vi "ZK_TriggerMouse.vi"(8 "Cluster 3":cluster{"X1":i32, "Y1":i32, "X2":i32, "Y2":i32}={"X1"=1479, "Y1"=207, "X2"=1532, "Y2"=259}, 10 "Result":T1={"A_Row"=2, "A_Col"=0, "B_Row"=1, "B_Col"=0}) -> ()   [LabVIEW 2018]
uses:
  <vilib>/Utility/error.llb/DialogType.ctl
  C:/Users/rshang/Desktop/LabVIEWZOOKEPPER_V2/ClassLibrary_ZK.dll
  ClassLibrary_ZK.dll
panel:
  out "String 2":string
  out "String":string
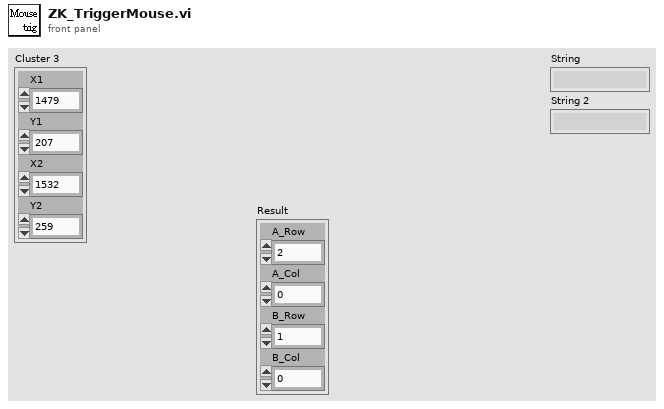
[diagram p1: front panel]
types:
  T1 = cluster{"A_Row":i32, "A_Col":i32, "B_Row":i32, "B_Col":i32}
  T2 = typedef "DialogType.ctl" = u16
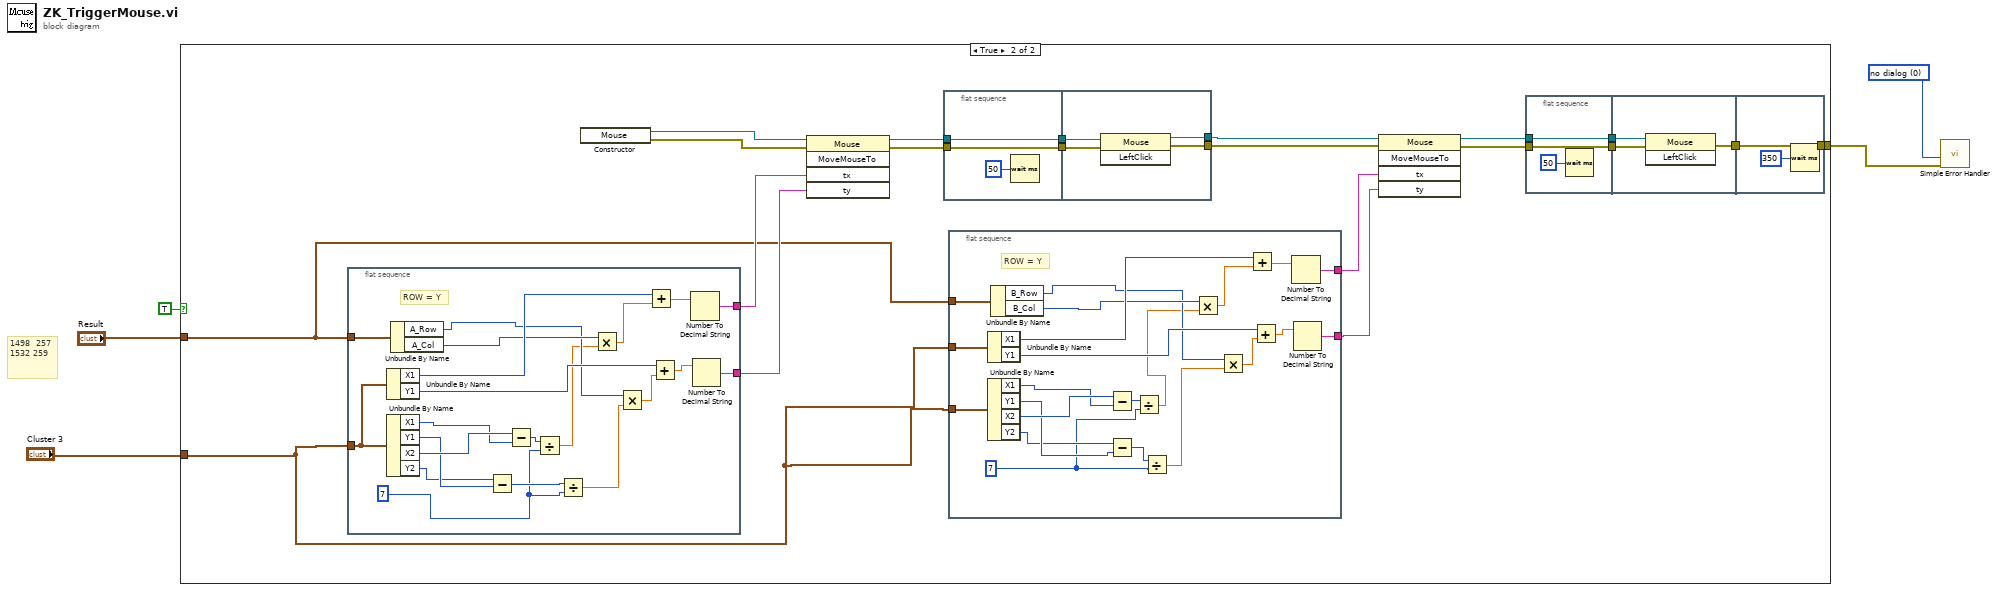
[diagram p0: block diagram]
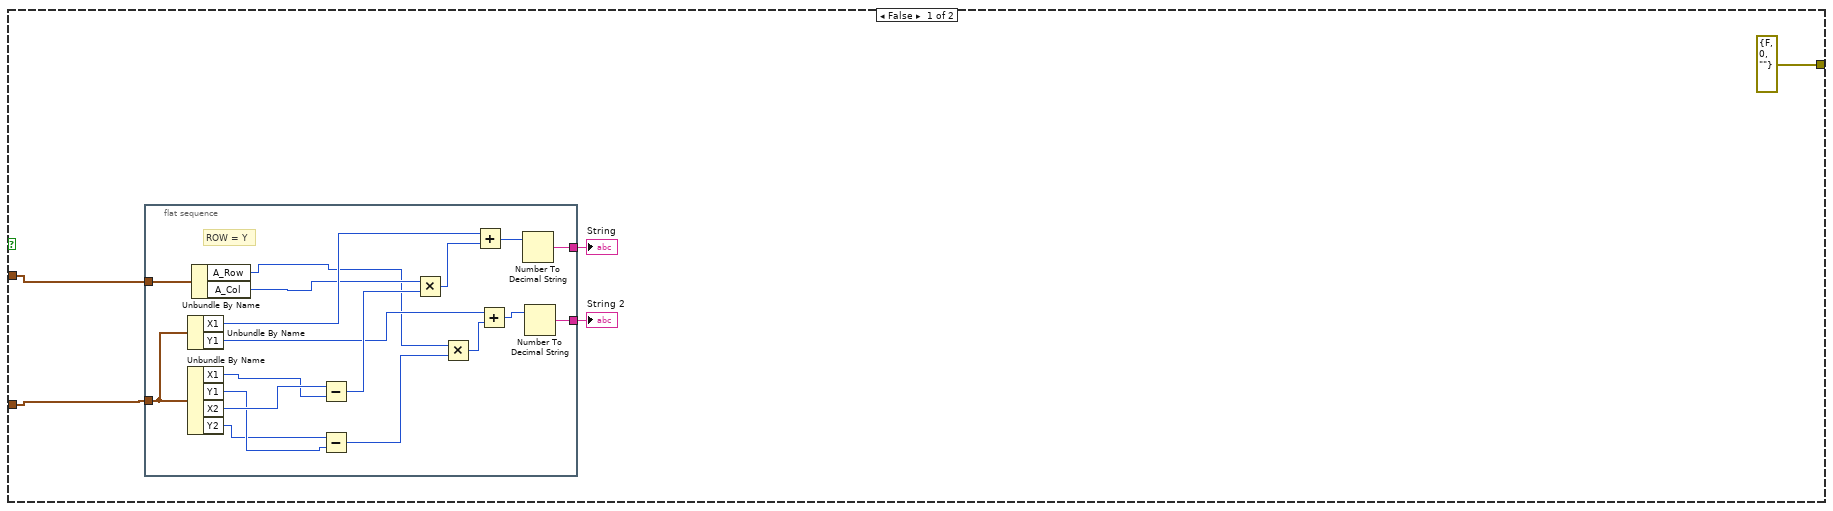
[diagram p2: hidden frame]
diagram:
  w1 = T2 0 items=["no dialog", "OK message", "continue or stop message", "OK message + warnings", "continue/stop + warnings"] ("type of dialog (OK msg:1)")
  # "1498  257 \n1532 259"
  n1 = case shown="True" TRUE {
    tunnel: "Result" -> [w10 w38]
    tunnel: "Cluster 3" -> [w9 w35]
    tunnel: [errorcluster {"status"=FALSE, "code"=0, "source"=""} ("error out") w30] -> w2
    frame False {
      n2 = flat-sequence {
        tunnel: [w16] -> w7
        tunnel: [w15] -> w8
        tunnel: w10 -> [w12]
        tunnel: w9 -> [w11]
        frame #0 {
          # "ROW = Y"
          n3 = Unbundle By Name(w11) -> ("X1"=w24:i32, "Y1"=w21:i32)
          n4 = Unbundle By Name(w11) -> ("X1"=w27:i32, "Y1"=w26:i32, "X2"=w28:i32, "Y2"=w25:i32)
          n5 = Unbundle By Name(w12) -> ("A_Row"=w13:i32, "A_Col"=w14:i32)
          n6 = Subtract(x=w28, y=w27) -> (x-y=w23:i32)
          n7 = Subtract(x=w25, y=w26) -> (x-y=w20:i32)
          n8 = Multiply(x=w14, y=w23) -> (x*y=w22:i32)
          n9 = Multiply(x=w13, y=w20) -> (x*y=w19:i32)
          n10 = Add(x=w24, y=w22) -> (x+y=w18:i32)
          n11 = Add(x=w21, y=w19) -> (x+y=w17:i32)
          n12 = Number To Decimal String(number=w18) -> (decimal integer string=w15:string)  [unwired: 1 in]
          n13 = Number To Decimal String(number=w17) -> (decimal integer string=w16:string)  [unwired: 1 in]
        }
      }
      "String" <- w8
      "String 2" <- w7
    }
    frame True {
      n14 = flat-sequence {
        tunnel: [w95] -> w46
        tunnel: [w94] -> w45
        tunnel: w38 -> [w91]
        tunnel: w35 -> [w90]
        frame #0 {
          w86 = 7 ("y")
          # "ROW = Y"
          n15 = Unbundle By Name(w90) -> ("X1"=w101:i32, "Y1"=w99:i32)
          n16 = Unbundle By Name(w90) -> ("X1"=w104:i32, "Y1"=w103:i32, "X2"=w105:i32, "Y2"=w102:i32)
          n17 = Unbundle By Name(w91) -> ("A_Row"=w92:i32, "A_Col"=w93:i32)
          n18 = Subtract(x=w102, y=w103) -> (x-y=w87:i32)
          n19 = Subtract(x=w105, y=w104) -> (x-y=w89:i32)
          n20 = Divide(x=w89, y=w86) -> (x/y=w88:dbl)
          n21 = Divide(x=w87, y=w86) -> (x/y=w85:dbl)
          n22 = Multiply(x=w93, y=w88) -> (x*y=w100:dbl)
          n23 = Multiply(x=w92, y=w85) -> (x*y=w98:dbl)
          n24 = Add(x=w101, y=w100) -> (x+y=w97:dbl)
          n25 = Add(x=w99, y=w98) -> (x+y=w96:dbl)
          n26 = Number To Decimal String(number=w97) -> (decimal integer string=w94:string)  [unwired: 1 in]
          n27 = Number To Decimal String(number=w96) -> (decimal integer string=w95:string)  [unwired: 1 in]
        }
      }
      n28 = constructor class="Mouse"() -> (reference out=w48:refnum<k24>, error out=w47:errorcluster)  [unwired: 3 in, 1 out]
      n29 = invoke class="Mouse" method="MoveMouseTo"(reference=w48, error in=w47, "tx"=w45, "ty"=w46) -> (reference out=w44:refnum<k24>, error out=w43:errorcluster)  [unwired: 1 in, 3 out]
      n30 = flat-sequence {
        tunnel: w43 -> [w58]
        tunnel: w44 -> [w59]
        tunnel: [w59] -> w34
        tunnel: [w58] -> w33
        tunnel: [w61] -> w42
        tunnel: [w60] -> w40
        tunnel: w34 -> [w63]
        tunnel: w33 -> [w62]
        frame #0 {
          n31 = Wait (ms)(milliseconds to wait=u32 50) -> ()  [unwired: 1 out]
        }
        frame #1 {
          n32 = invoke class="Mouse" method="LeftClick"(reference=w63, error in=w62) -> (reference out=w61:refnum<k24>, error out=w60:errorcluster)  [unwired: 1 in, 1 out]
        }
      }
      n33 = flat-sequence {
        tunnel: [w74] -> w36
        tunnel: [w73] -> w37
        tunnel: w38 -> [w70]
        tunnel: [w69] -> _
        tunnel: w35 -> [w69]
        tunnel: w35 -> [_]
        frame #0 {
          w65 = 7 ("y")
          # "ROW = Y"
          n34 = Unbundle By Name(w69) -> ("X1"=w80:i32, "Y1"=w78:i32)
          n35 = Unbundle By Name(w69) -> ("X1"=w83:i32, "Y1"=w82:i32, "X2"=w84:i32, "Y2"=w81:i32)
          n36 = Unbundle By Name(w70) -> ("B_Row"=w71:i32, "B_Col"=w72:i32)
          n37 = Subtract(x=w84, y=w83) -> (x-y=w68:i32)
          n38 = Subtract(x=w81, y=w82) -> (x-y=w66:i32)
          n39 = Divide(x=w68, y=w65) -> (x/y=w67:dbl)
          n40 = Divide(x=w66, y=w65) -> (x/y=w64:dbl)
          n41 = Multiply(x=w72, y=w67) -> (x*y=w79:dbl)
          n42 = Multiply(x=w71, y=w64) -> (x*y=w77:dbl)
          n43 = Add(x=w80, y=w79) -> (x+y=w76:dbl)
          n44 = Add(x=w78, y=w77) -> (x+y=w75:dbl)
          n45 = Number To Decimal String(number=w76) -> (decimal integer string=w73:string)  [unwired: 1 in]
          n46 = Number To Decimal String(number=w75) -> (decimal integer string=w74:string)  [unwired: 1 in]
        }
      }
      n47 = invoke class="Mouse" method="MoveMouseTo"(reference=w42, error in=w40, "tx"=w37, "ty"=w36) -> (reference out=w41:refnum<k24>, error out=w39:errorcluster)  [unwired: 1 in, 3 out]
      n48 = flat-sequence {
        tunnel: w39 -> [w50]
        tunnel: w41 -> [w51]
        tunnel: [w51] -> w32
        tunnel: [w50] -> w31
        tunnel: w32 -> [w54]
        tunnel: w31 -> [w53]
        tunnel: [w52] -> w29
        tunnel: [w56] -> w30
        tunnel: w29 -> [w56]
        frame #0 {
          n49 = Wait (ms)(milliseconds to wait=u32 50) -> ()  [unwired: 1 out]
        }
        frame #1 {
          n50 = invoke class="Mouse" method="LeftClick"(reference=w54, error in=w53) -> (error out=w52:errorcluster)  [unwired: 1 in, 2 out]
        }
        frame #2 {
          n51 = Wait (ms)(milliseconds to wait=u32 350) -> ()  [unwired: 1 out]
        }
      }
    }
  }
  n52 = call <vilib>:"Simple Error Handler.vi"("type of dialog (OK msg:1)"=w1, "error in (no error)"=w2) -> ()  [unwired: 3 in, 5 out]
